vi "Dynamic Lock 2k.vi"(9 "Page Selection":T1=enum."1.B0-1.CF [13]", 11 "PN532 COM Port":refnum<visa-resource-name>) -> (0 "Error out":errorcluster, 2 "Succeeded":bool)   [LabVIEW 2012, in "NFC Driver.lvlib"]
uses:
  NFC Driver.lvlib
  Typedef/Dynamic Lock Page Section 2K.ctl
panel:
  out "PN532 COM Port Out":refnum<visa-resource-name>
  out "result string":string
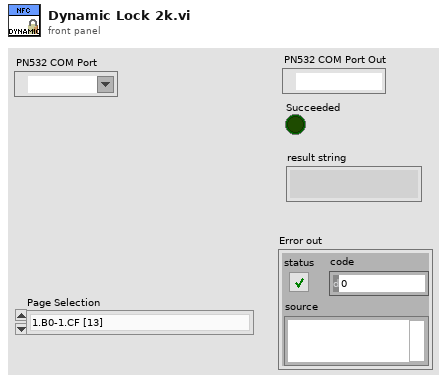
[diagram p1: front panel]
types:
  T1 = typedef "NFC Driver.lvlib/Dynamic Lock Page Section 2K.ctl" = enum16{"0.10-0.2F [0]", "0.30-0.4F [1]", "0.50-0.6F [2]", "0.70-0.8F [3]", "0.90-0.AF [4]", "0.B0-0.CF [5]", "0.D0-0.EF [6]", "0.F0-1.0F [7]", "1.10-1.2F [8]", "1.30-1.4F [9]", "1.50-1.6F [10]", "1.70-1.8F [11]", "1.90-1.AF [12]", "1.B0-1.CF [13]", "1.D0-1.DF [14]"}
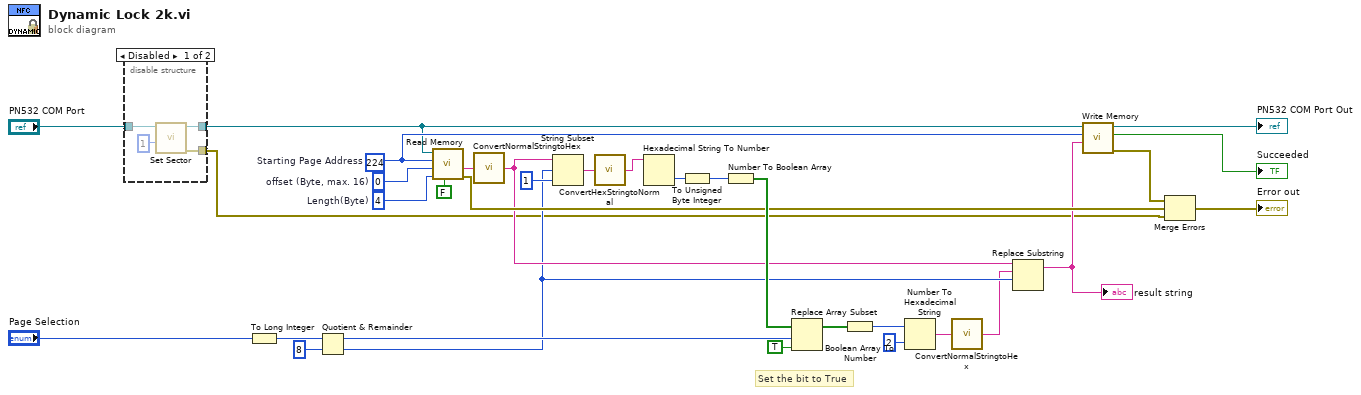
[diagram p0: block diagram]
diagram:
  w13 = 0  # offset (Byte, max. 16)
  w30 = 4  # Length(Byte)
  w11 = 224  # Starting Page Address
  # "Set the bit to True"
  n1 = disable-structure shown="Disabled" {
    disable-tunnel: "PN532 COM Port" -> [w36 w37]
    disable-tunnel: [w35 w37] -> w5
    disable-tunnel: [w33 _] -> w4
    frame Disabled {
      n2 = call "Set Sector.vi"("Numeric"=1, "PN532 COM Port"=w36) -> ("Error Out"=w33:errorcluster, "PN532 COM out"=w35:refnum<visa-resource-name>)  [unwired: 8 in]
    }
    frame Enabled {
    }
  }
  n3 = To Long Integer(number="Page Selection") -> (32bit integer=w19:i32)
  n4 = Quotient & Remainder(x=w19, y=8) -> (x-y*floor(x/y)=w20:i32, floor(x/y)=w10:i32)
  n5 = call "Read Memory.vi"("Reverse Output[F]"=FALSE, "length (Byte, max. 16)"=w30, "offset (Byte, max. 16)"=w13, "Page Address"=w11, "PN532 COM Port"=w5) -> ("error out"=w24:errorcluster, "Selected substring (HEX)"=w1:string)  [unwired: 2 in, 3 out]
  n6 = call "ConvertNormalStringtoHex.vi"("Normal String"=w1) -> ("Hex String"=w12:string)
  n7 = String Subset(string=w12, offset (0)=w10, length (rest)=1 ("length (rest)")) -> (substring=w16:string)
  n8 = call "ConvertHexStringtoNormal.vi"("Hex String"=w16) -> ("Normal String"=w15:string)
  n9 = Hexadecimal String To Number(string=w15) -> (number=w29:u32)  [unwired: 2 in, 1 out]
  n10 = To Unsigned Byte Integer(number=w29) -> (unsigned 8bit integer=w17:u8)
  n11 = Number To Boolean Array(number=w17) -> (Boolean array=w28:bool[])
  n12 = Replace Array Subset(array=w28, new element=TRUE ("new element/subarray"), index=w20) -> (w23:bool[])
  n13 = Boolean Array To Number(Boolean array=w23) -> (number=w27:u32)
  n14 = Number To Hexadecimal String(1:i16 2 ("width (-)"), 2:w27) -> (0:w9:string)
  n15 = call "ConvertNormalStringtoHex.vi"("Normal String"=w9) -> ("Hex String"=w7:string)
  n16 = Replace Substring(3:w10, 4:w7, 5:w12) -> (1:w8:string)  [unwired: 1 in, 1 out]
  "result string" <- w8
  n17 = call "Write Memory.vi"("Data to write (HEX, max 16 bytes)"=w8, "Page Address"=w11, "PN532 COM Port"=w5) -> ("Error Out"=w25:errorcluster, "Succesful?"=→"Succeeded":bool, "PN532 COM Port Out"=→"PN532 COM Port Out":refnum<visa-resource-name>)  [unwired: 6 in]
  n18 = Merge Errors(w25, w24, w4) -> (→"Error out":errorcluster)
